vi "Create Client Hello.vi"(8 "error in (no error)":errorcluster, 11 "TCPMessaging in":refnum<class "TCPMessaging.lvclass">) -> (0 "error out":errorcluster, 2 "TcpClientHello":T1, 3 "TCPMessaging out":refnum<class "TCPMessaging.lvclass">)   [LabVIEW 2020, in "Vecto.lvlib" / "TCPMessaging.lvclass"]
uses:
  TCPMessaging.lvclass
  lv-volatus/messages/TcpClientHello/Data.ctl
  TCPMessaging.lvclass/TCPMessaging.ctl
  lv-volatus/messages/TcpClientHello/TcpClientHello.lvlib
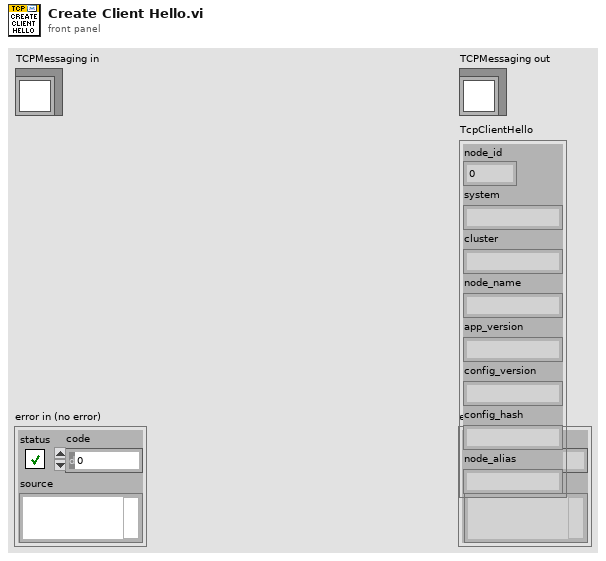
[diagram p1: front panel]
types:
  T1 = typedef "TcpClientHello.lvlib/Data.ctl" = cluster{"node_id":u32, "system":string, "cluster":string, "node_name":string, "app_version":string, "config_version":string, "config_hash":string, "node_alias":string}
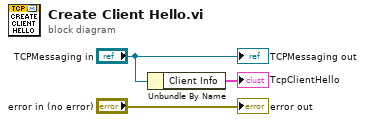
[diagram p0: block diagram]
diagram:
  n1 = Unbundle By Name("TCPMessaging in") -> ("Client Info"=→"TcpClientHello":T1)
  "error out" <- "error in (no error)"
  "TCPMessaging out" <- "TCPMessaging in"
